vi "practica 2.vi"() -> ()   [LabVIEW 2016]
panel:
  out "XY Graph":cluster{"X":dbl[], "Y":dbl[]}[](graph)
  out "output variable":dbl
  out "alcance":dbl
  out "tiempo":i32
  in  "velocidad inicial":dbl
  in  "cateto adyacente":dbl
  in  "cateto opuesto":dbl
  in  "stop":bool
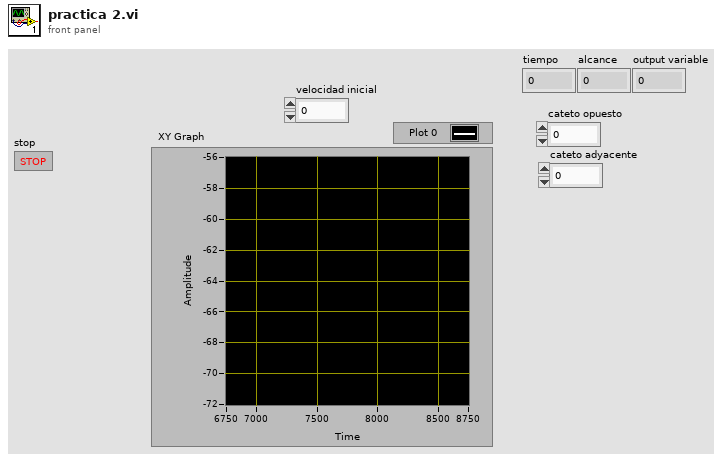
[diagram p1: front panel]
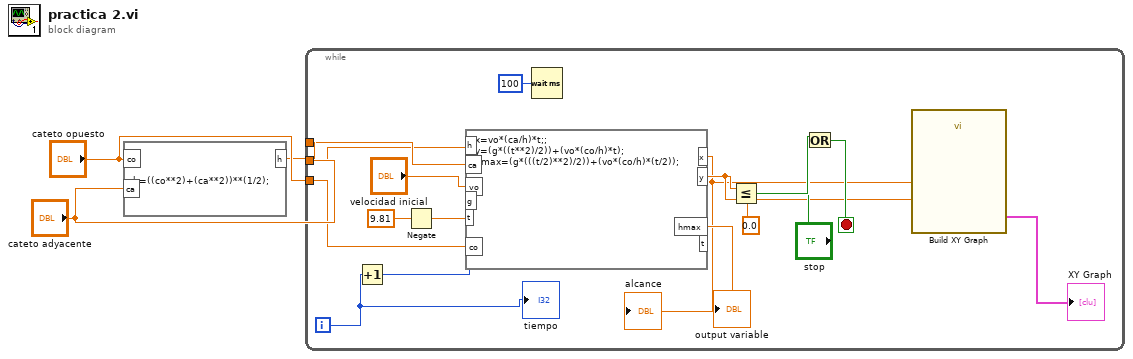
[diagram p0: block diagram]
diagram:
  n1 = formula code="h=((co**2)+(ca**2))**(1/2);"("co"="cateto opuesto", "ca"="cateto adyacente") -> ("h"=w1:dbl)
  n2 = while {
    tunnel: "cateto opuesto" -> [w16]
    tunnel: "cateto adyacente" -> [w17]
    tunnel: w1 -> [w18]
    i -> [w9]
    stop <- w12 stop-if-true
    n3 = Increment(x=w9) -> (x+1=w11:i32)
    n4 = Negate(x=9.81) -> (-x=w8:dbl)
    n5 = formula code="x=vo*(ca/h)*t;;\ny=(g*((t**2)/2))+(vo*(co/h)*t);\nhmax=(g*(((t/2)**2)/2))+(vo*(co/h)*(t/2));"("t"=w11, "vo"="velocidad inicial", "ca"=w18, "co"=w16, "h"=w17, "g"=w8) -> ("y"=w6:dbl, "hmax"=→"output variable":dbl, "x"=w4:dbl)  [unwired: 1 out]
    "alcance" <- w4
    n6 = Wait (ms)(milliseconds to wait=u32 100) -> ()  [unwired: 1 out]
    n7 = Less Or Equal?(x=w6, y=0.0) -> (x <= y?=w14:bool)
    n8 = Or(x=w14, y="stop") -> (x .or. y?=w12:bool)
    n9 = call "Build XY Graph"("Y Input"=w6, "X Input"=w4) -> ("XY Graph"=→"XY Graph":cluster{"X":dbl[], "Y":dbl[]}[])  [unwired: 8 in, 1 out]
    "tiempo" <- w9
  }
